vi "Poll.Selection.vi"(6 "Existing Names":string[](array[string]), 7 "Name":string, 8 "error in (no error)":errorcluster, 9 "Already Used":T2[](array[typedef]), 10 "Selected Channels":T4, 11 "Node Ptr":T3 format="%.0x") -> (0 "error out":errorcluster, 1 "Cancel out":bool, 2 "Selected Channels":T4, 3 "Node Ptr out":T3 format="%.0x", 5 "Name out":string)   [LabVIEW 2019, in "Diagnostics Addon System Explorer.lvlib"]
uses:
  Diagnostics Addon System Explorer.lvlib
  NationalInstruments.VeriStand.SystemStorageUI
  NationalInstruments.VeriStand.SystemStorage
  <vilib>/NI VeriStand/Custom Device API/Custom Device API.lvlib
  NationalInstruments.VeriStand.SystemDefinitionAPI
  Types/Poll.LinkedNode.ctl
  Shared/SubVIs/Constants.vi
  Shared/Diagnostics Addon Shared.lvlib
  NationalInstruments.VeriStand
  <vilib>/NI VeriStand/Custom Device API/Custom Device Item Ref.ctl
  Shared/Types/DPID.Rate.ctl
  Types/Poll.Settings.ctl
panel:
  in  "Speed":T1
  in  "Cancel":bool
  in  "Apply":bool
  in  "Select":refnum<k24>(container)
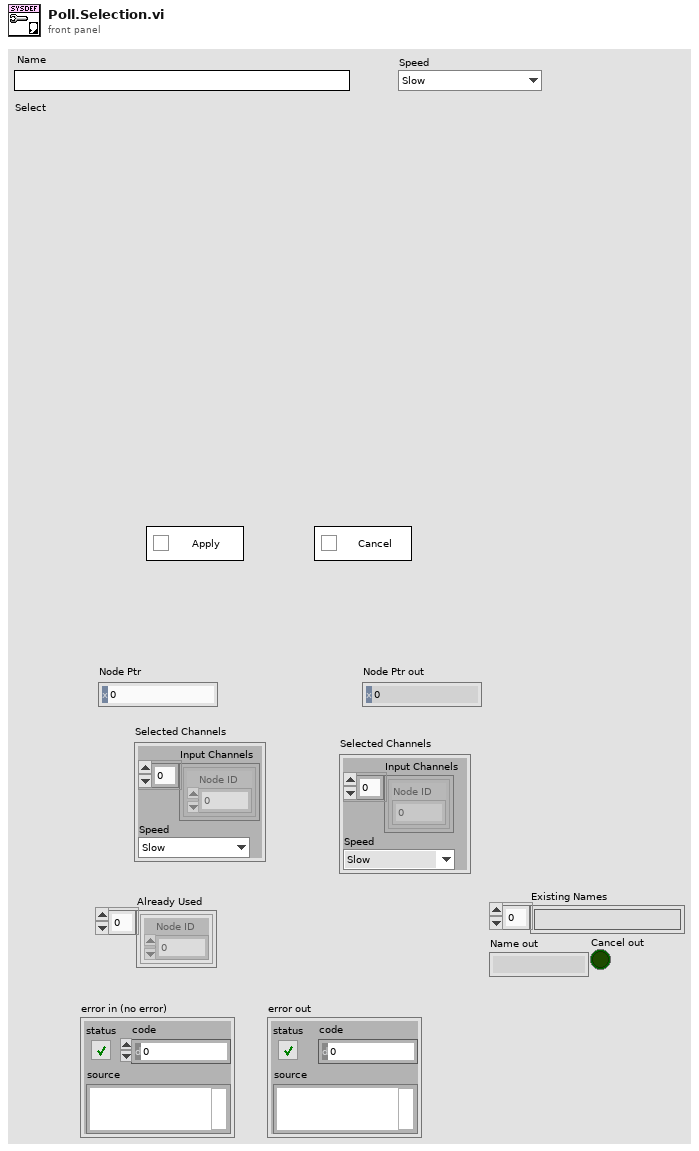
[diagram p1: front panel]
types:
  T1 = typedef "Diagnostics Addon Shared.lvlib/DPID.Rate.ctl" = enum16{"Slow", "Medium", "Fast"}
  T2 = typedef "Diagnostics Addon System Explorer.lvlib/Poll.LinkedNode.ctl" = cluster{"Node ID":u64}
  T3 = typedef "Custom Device API.lvlib/Custom Device Item Ref.ctl" = u64
  T4 = typedef "Diagnostics Addon System Explorer.lvlib/Poll.Settings.ctl" = cluster{"Input Channels":T2[], "Speed":T1}
  T5 = typedef "Custom Device API.lvlib/Custom Device Pointer.ctl" = refnum<k24>
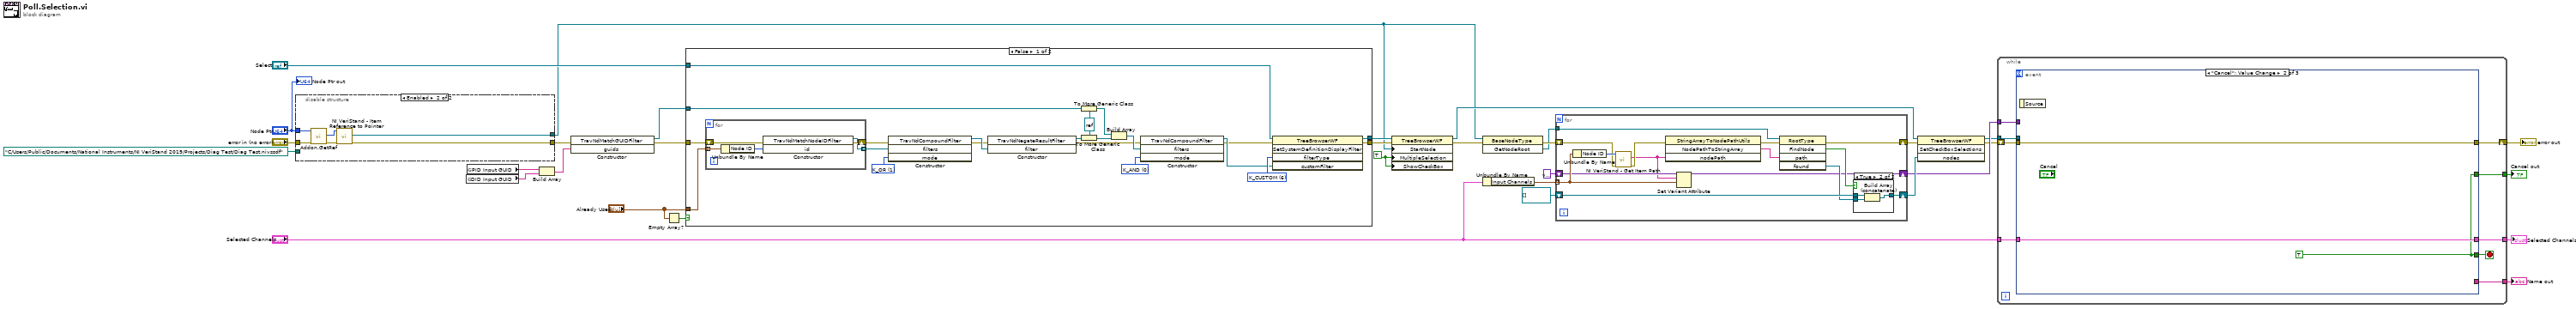
[diagram p0: block diagram]
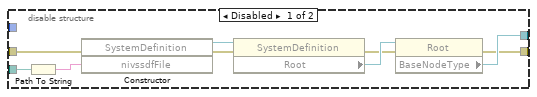
[diagram p2: hidden frame]
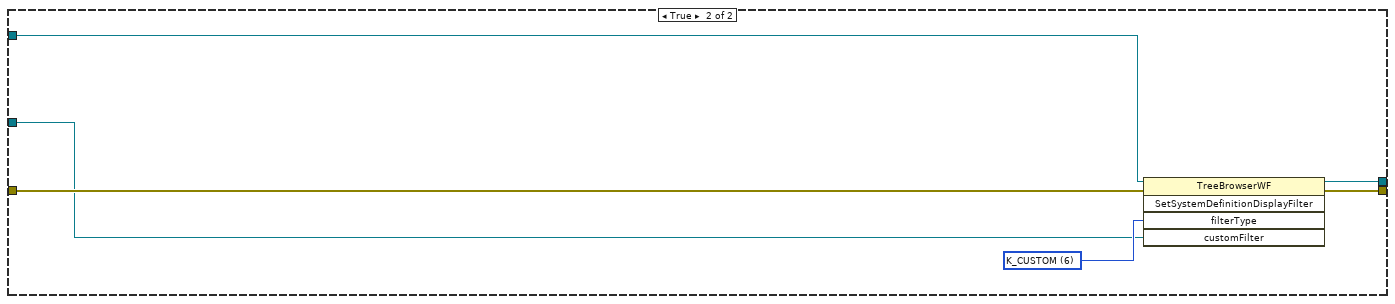
[diagram p3: hidden frame]
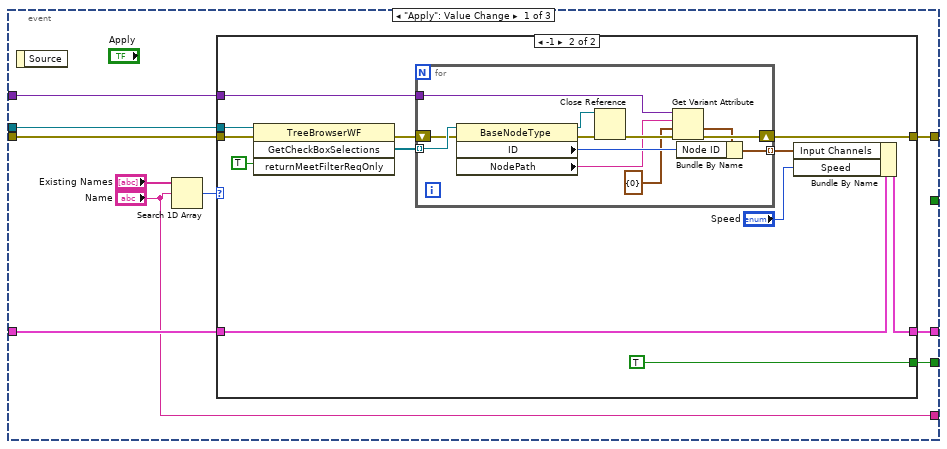
[diagram p5: hidden frame]
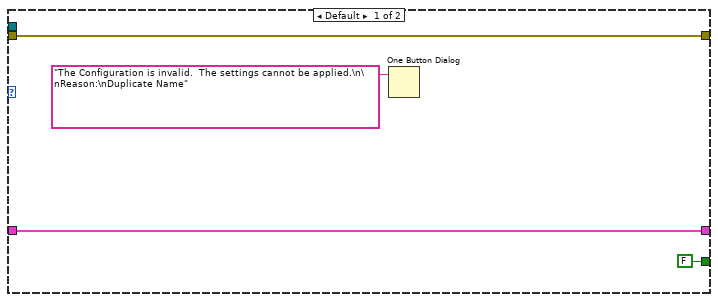
[diagram p6: hidden frame]
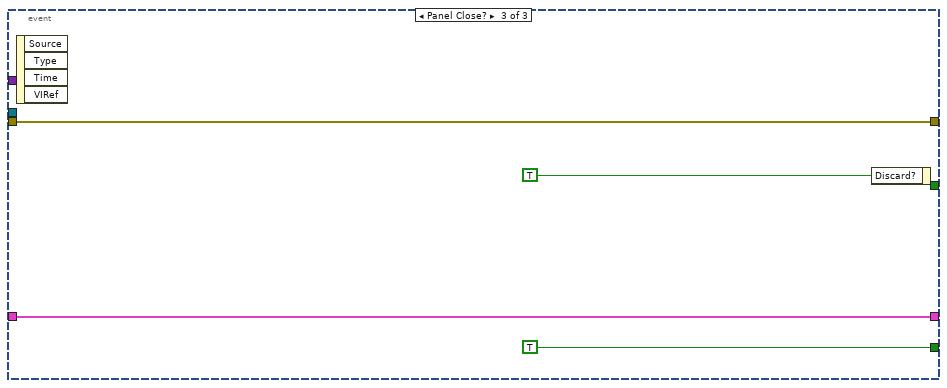
[diagram p7: hidden frame]
diagram:
  w29 = TRUE ("MultipleSelection")
  n1 = disable-structure shown="Enabled" {
    disable-tunnel: path "C:/Users/Public/Documents/National Instruments/NI VeriStand 2019/Projects/Diag Test/Diag Test.nivssdf" ("path") -> [w41 _]
    disable-tunnel: [w37 w48] -> w15
    disable-tunnel: "error in (no error)" -> [w35 w45]
    disable-tunnel: [w34 w47] -> w13
    disable-tunnel: "Node Ptr" -> [_ w46]
    frame Disabled {
      n2 = Path To String(path=w41) -> (string=w42:string)
      n3 = constructor class="SystemDefinition"(error in=w35, "nivssdfFile"=w42) -> (reference out=w40:refnum<k24>, error out=w39:errorcluster)  [unwired: 2 in, 2 out]
      n4 = property class="SystemDefinition"(reference=w40, error in=w39) -> (error out=w36:errorcluster, "Root"=w38:refnum<k24>)  [unwired: 1 out]
      n5 = property class="Root"(reference=w38, error in=w36) -> (error out=w34:errorcluster, "BaseNodeType"=w37:refnum<k24>)  [unwired: 1 out]
    }
    frame Enabled {
      n6 = call "Addon.GetRef.vi"("error in (no error)"=w45, "Node Ptr"=w46) -> ("error out"=w44:errorcluster, "Addon Ref"=w43:T3)  [unwired: 7 in, 1 out]
      n7 = call <vilib>:"NI VeriStand - Item Reference to Pointer.vi"("error in (no error)"=w44, "Item Ref in"=w43) -> ("error out"=w47:errorcluster, "Node Pointer"=w48:T5)  [unwired: 6 in, 2 out]
    }
  }
  n8 = global read "Constants.vi" "DID Input GUID"() -> (w5:string)
  n9 = global read "Constants.vi" "PID Input GUID"() -> (w6:string)
  n10 = Build Array(w6, w5) -> (w4:string[])
  n11 = constructor class="TravNdMatchGUIDFilter"(error in=w13, "guids"=w4) -> (reference out=w8:refnum<k24>, error out=w10:errorcluster)  [unwired: 2 in, 2 out]
  n12 = Empty Array?(array="Already Used") -> (empty?=w7:bool)
  n13 = case shown="False" w7 {
    tunnel: [w68 w77] -> w24
    tunnel: [w67 w76] -> w23
    tunnel: "Select" -> [w66 w78]
    tunnel: w10 -> [w64 w79]
    tunnel: "Already Used" -> [w62 _]
    tunnel: w8 -> [w51 w75]
    frame False {
      w49 = refnum<k24> refnum
      w56 = 1 items=["K_AND", "K_OR"] ("mode")
      w59 = 0 items=["K_AND", "K_OR"] ("mode")
      w69 = u8 6 items=["K_CHAN_R", "K_CHAN_W", "K_CHAN_RW", "K_CHAN_VOLT", "K_CHAN_FAULT", "K_ALL", "K_CUSTOM", "K_CHAN_R_VIS", "K_CHAN_W_VIS", "K_CHAN_RW_VIS", "K_CHAN_VOLT_VIS", "K_CHAN_FAULT_VIS", "K_WAVE", "K_WAVE_VIS", "K_WAVE_DBL", "K_WAVE_CDB", "K_WAVE_DBL_VIS", "K_WAVE_CDB_VIS"] ("filterType")
      n14 = for {
        tunnel: [w72] -> w55 mode=indexing
        shift-right: [w74] -> w53
        shift-left: w64 -> [w73]
        tunnel: w62 -> [w71] mode=indexing
        n15 = Unbundle By Name(w71) -> ("Node ID"=w70:u64)
        n16 = constructor class="TravNdMatchNodeIDFilter"(error in=w73, "id"=w70) -> (reference out=w72:refnum<k24>, error out=w74:errorcluster)  [unwired: 2 in, 2 out]
      }
      n17 = constructor class="TravNdCompoundFilter"(error in=w53, "filters"=w55, "mode"=w56) -> (reference out=w54:refnum<k24>, error out=w52:errorcluster)  [unwired: 2 in, 3 out]
      n18 = constructor class="TravNdNegateResultFilter"(error in=w52, "filter"=w54) -> (reference out=w58:refnum<k24>, error out=w57:errorcluster)  [unwired: 2 in, 2 out]
      n19 = To More Generic Class(target class=w49, reference=w51) -> (generic class reference=w50:refnum<k24>)
      n20 = To More Generic Class(target class=w49, reference=w58) -> (generic class reference=w61:refnum<k24>)
      n21 = Build Array(w50, w61) -> (w60:refnum<k24>[])
      n22 = constructor class="TravNdCompoundFilter"(error in=w57, "filters"=w60, "mode"=w59) -> (reference out=w65:refnum<k24>, error out=w63:errorcluster)  [unwired: 2 in, 3 out]
      n23 = invoke class="TreeBrowserWF" method="SetSystemDefinitionDisplayFilter"(reference=w66, error in=w63, "filterType"=w69, "customFilter"=w65) -> (reference out=w67:refnum<k24>, error out=w68:errorcluster)  [unwired: 1 in, 3 out]
    }
    frame True {
      w80 = u8 6 items=["K_CHAN_R", "K_CHAN_W", "K_CHAN_RW", "K_CHAN_VOLT", "K_CHAN_FAULT", "K_ALL", "K_CUSTOM", "K_CHAN_R_VIS", "K_CHAN_W_VIS", "K_CHAN_RW_VIS", "K_CHAN_VOLT_VIS", "K_CHAN_FAULT_VIS", "K_WAVE", "K_WAVE_VIS", "K_WAVE_DBL", "K_WAVE_CDB", "K_WAVE_DBL_VIS", "K_WAVE_CDB_VIS"] ("filterType")
      n24 = invoke class="TreeBrowserWF" method="SetSystemDefinitionDisplayFilter"(reference=w78, error in=w79, "filterType"=w80, "customFilter"=w75) -> (reference out=w76:refnum<k24>, error out=w77:errorcluster)  [unwired: 1 in, 3 out]
    }
  }
  n25 = property class="TreeBrowserWF"(reference=w23, error in=w24, "StartNode"=w15, "MultipleSelection"=w29, "ShowCheckBox"=w29) -> (reference out=w26:refnum<k24>, error out=w25:errorcluster)
  n26 = invoke class="BaseNodeType" method="GetNodeRoot"(reference=w15, error in=w25) -> (error out=w33:errorcluster, "GetNodeRoot"=w32:refnum<k24>)  [unwired: 1 in, 1 out]
  n27 = Unbundle By Name("Selected Channels") -> ("Input Channels"=w3:T2[])
  n28 = for {
    shift-right: [w92] -> w28
    shift-left: w33 -> [w83]
    tunnel: w3 -> [w87] mode=indexing
    tunnel: w32 -> [w95]
    shift-right: [w89] -> w30
    shift-left: refnum<k24>[] [] -> [w90]
    shift-right: [w85] -> w20
    shift-left: variant -> [w86]
    n29 = Unbundle By Name(w87) -> ("Node ID"=w84:u64)
    n30 = call <vilib>:"NI VeriStand - Get Item Path.vi"("error in (no error)"=w83, "Item Ref in"=w84) -> ("error out"=w82:errorcluster, "Path"=w81:string)  [unwired: 6 in, 2 out]
    n31 = invoke class="StringArrayToNodePathUtils" method="NodePathToStringArray"(error in=w82, "nodePath"=w81) -> (error out=w93:errorcluster, "NodePathToStringArray"=w94:string[])  [unwired: 2 in, 2 out]
    n32 = Set Variant Attribute(Variant=w86, name=w81, value=w87) -> (Variant out=w85:variant)  [unwired: 1 in, 2 out]
    n33 = invoke class="RootType" method="FindNode"(reference=w95, error in=w93, "path"=w94) -> (error out=w92:errorcluster, "FindNode"=w91:bool, "found"=w88:refnum<k24>)  [unwired: 2 in, 2 out]
    n34 = case shown="True" w91 {
      tunnel: w90 -> [w96 w99]
      tunnel: [w96 w97] -> w89
      tunnel: w88 -> [_ w98]
      frame False {
      }
      frame True {
        n35 = Build Array (concatenate)(w99, w98) -> (w97:refnum<k24>[])
      }
    }
  }
  n36 = invoke class="TreeBrowserWF" method="SetCheckBoxSelections"(reference=w26, error in=w28, "nodes"=w30) -> (reference out=w18:refnum<k24>, error out=w19:errorcluster)  [unwired: 1 in, 2 out]
  n37 = while {
    tunnel: [w108] -> w22
    tunnel: w20 -> [w107]
    tunnel: w18 -> [w105]
    shift-right: [w104] -> w17
    shift-left: w19 -> [w106]
    tunnel: "Selected Channels" -> [w102]
    tunnel: [w101] -> w2
    tunnel: [w100] -> w1
    stop <- w103 stop-if-true
    n38 = event shown="[1] \"Cancel\": Value Change" {
      selector: _ -> [_ _ _]
      dyn-events: _ -> [_ _ _]
      timeout: _ -> [_ _ _]
      tunnel: [w113 w149 w153] -> w108
      tunnel: w107 -> [w118 _ _]
      tunnel: w106 -> [w117 w148 w152]
      tunnel: w105 -> [w116 _ _]
      tunnel: [w115 w148 w152] -> w104
      tunnel: [w110 w147 TRUE ("Boolean")] -> w103
      tunnel: w102 -> [w114 w149 w153]
      tunnel: ["Name" _ _] -> w101
      tunnel: [_ w147 _] -> w100
      event "Apply": Value Change {
        n39 = event-data() -> ()  [unwired: 1 in, 1 out]
        n40 = Search 1D Array(1D array="Existing Names", element="Name") -> (index of element=w111:i32)  [unwired: 1 in]
        n41 = case shown="-1" w111 {
          tunnel: w118 -> [_ w131]
          tunnel: w117 -> [w121 w130]
          tunnel: w116 -> [_ w129]
          tunnel: [w121 w128] -> w115
          tunnel: w114 -> [w122 w127]
          tunnel: [w122 w125] -> w113
          tunnel: [FALSE ("Boolean") TRUE ("Boolean")] -> w110
          frame Default {
            n42 = One Button Dialog(message="The Configuration is invalid.  The settings cannot be applied.\n\nReason:\nDuplicate Name") -> ()  [unwired: 1 in, 1 out]
          }
          frame -1 {
            n43 = invoke class="TreeBrowserWF" method="GetCheckBoxSelections"(reference=w129, error in=w130, "returnMeetFilterReqOnly"=TRUE) -> (error out=w134:errorcluster, "GetCheckBoxSelections"=w133:refnum<k24>[])  [unwired: 1 in, 2 out]
            n44 = for {
              tunnel: w133 -> [w146] mode=indexing
              shift-right: [w142] -> w128
              shift-left: w134 -> [w145]
              tunnel: [w143] -> w126 mode=indexing
              tunnel: w131 -> [w141]
              n45 = property class="BaseNodeType"(reference=w146, error in=w145) -> (reference out=w137:refnum<k24>, error out=w139:errorcluster, "ID"=w144:u64, "NodePath"=w136:string)
              n46 = Close Reference(reference=w137, error in (no error)=w139) -> (error out=w138:errorcluster)
              n47 = Get Variant Attribute(Variant=w141, name=w136, default value (empty Variant)=T2 {"Node ID"=0} ("MonitoredChannelSettings"), error in=w138) -> (value=w140:T2, error out=w142:errorcluster)  [unwired: 2 out]
              n48 = Bundle By Name(cluster=w140, "Node ID"=w144) -> (w143:T2)
            }
            n49 = Bundle By Name(cluster=w127, "Input Channels"=w126, "Speed"="Speed") -> (w125:T4)
          }
        }
      }
      event "Cancel": Value Change {
        w147 = TRUE ("Boolean")
        n50 = event-data() -> ()  [unwired: 1 in, 1 out]
      }
      event Panel Close? {
        n51 = event-data() -> ()  [unwired: 1 in, 4 out]
        n52 = event-data("Discard?"=TRUE) -> ()  [unwired: 1 in, 1 out]
      }
    }
  }
  "error out" <- w17
  "Selected Channels" <- w22
  "Name out" <- w2
  "Cancel out" <- w1
  "Node Ptr out" <- "Node Ptr"
